vi "LiftPIDSpeed.vi"(6 "joystick":dbl, 8 "right encoder":dbl, 9 "left encoder":dbl, 10 "Distance PID":T1={"proportional gain (Kc)"=1.0, "integral time (Ti, min)"=0.01, "derivative time (Td, min)"=0.0} {"derivative time (Td, min)" format="%.3f"; "integral time (Ti, min)" format="%.3f"; "proportional gain (Kc)" format="%.3f"}, 11 "Difference PID":T1={"proportional gain (Kc)"=1.0, "integral time (Ti, min)"=0.01, "derivative time (Td, min)"=0.0} {"derivative time (Td, min)" format="%.3f"; "integral time (Ti, min)" format="%.3f"; "proportional gain (Kc)" format="%.3f"}) -> (0 "Right Motor":dbl format="%.2f", 3 "Left Motor":dbl format="%.2f")   [LabVIEW 2014]
uses:
  <vilib>/addons/control/pid/pid.llb/PID (DBL).vi
  <vilib>/addons/control/pid/NI_PID_pid.lvlib
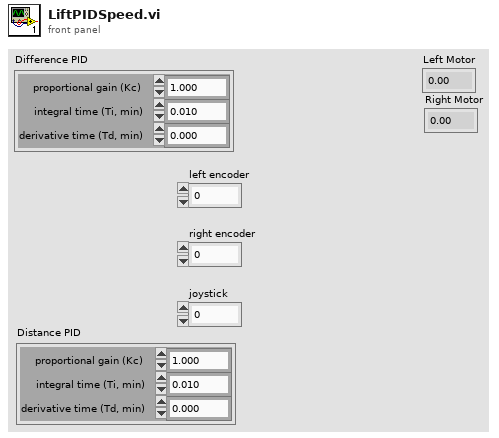
[diagram p1: front panel]
types:
  T1 = cluster{"proportional gain (Kc)":dbl, "integral time (Ti, min)":dbl, "derivative time (Td, min)":dbl}
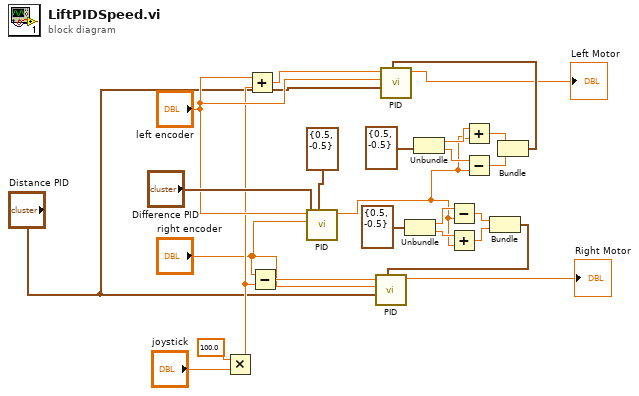
[diagram p0: block diagram]
diagram:
  n1 = Multiply(x=100.0, y="joystick") -> (x*y=w18:dbl)
  n2 = Add(x="left encoder", y=w18) -> (x+y=w21:dbl)
  n3 = Subtract(x="right encoder", y=w18) -> (x-y=w19:dbl)
  n4 = call-poly <vilib>:"PID.vi"("output range"=cluster{"output high":dbl, "output low":dbl} {"output high"=0.5, "output low"=-0.5}, "PID gains"="Difference PID", "process variable"="right encoder", "setpoint"="left encoder") -> ("output"=w6:dbl)  [unwired: 6 in, 1 out]
  n5 = Unbundle(cluster{"output high":dbl, "output low":dbl} {"output high"=0.5, "output low"=-0.5} ("output range")) -> ("output high"=w14:dbl, "output low"=w13:dbl)
  n6 = Unbundle(cluster{"output high":dbl, "output low":dbl} {"output high"=0.5, "output low"=-0.5} ("output range")) -> ("output high"=w8:dbl, "output low"=w7:dbl)
  n7 = Subtract(x=w14, y=w6) -> (x-y=w12:dbl)
  n8 = Add(x=w13, y=w6) -> (x+y=w11:dbl)
  n9 = Add(x=w8, y=w6) -> (x+y=w5:dbl)
  n10 = Subtract(x=w7, y=w6) -> (x-y=w4:dbl)
  n11 = Bundle(w12, w11) -> (w10:cluster{dbl, dbl})  [unwired: 1 in]
  n12 = call-poly <vilib>:"PID.vi"("output range"=w10, "PID gains"="Distance PID", "process variable"="right encoder", "setpoint"=w19) -> ("output"=→"Right Motor":dbl)  [unwired: 6 in, 1 out]
  n13 = Bundle(w5, w4) -> (w3:cluster{dbl, dbl})  [unwired: 1 in]
  n14 = call-poly <vilib>:"PID.vi"("output range"=w3, "PID gains"="Distance PID", "process variable"="left encoder", "setpoint"=w21) -> ("output"=→"Left Motor":dbl)  [unwired: 6 in, 1 out]
